vi "FPGA Main v0.2z.vi"() -> ()   [LabVIEW 2021]
uses:
  <vilib>/rvi/Emulation/niFpgaGetClockAttributes.vi
  <vilib>/rvi/Emulation/niFpgaSctlEmulationGetInTimedLoop.vi
  <vilib>/rvi/Emulation/niFpgaEmulationReportErrorSimple.vi
  <vilib>/rvi/eio/common/nirviEmuTemplateMethod_errors.vi
  <vilib>/rvi/Emulation/niFpgaCriticalErrorInLSC.vi
  <vilib>/eio/EIONode/EIONode.xnode
  <vilib>/rvi/FXPMathLib/FxpSub/XNode/nifxpmath_Sub.xnode
  <vilib>/rvi/FXPMathLib/sim/FxpSim.dll
panel:
  in  "DO 1":T1
  out "DI 2":T2
  out "DI 1":T3
  in  "Loop Time (ms)":u32=1 caption="Count(mSec)"
  in  "Stop Button":bool
  out "AI3":fxp<+/-,27,6> format="%.23g"
  out "AI2":fxp<+/-,27,6> format="%.23g"
  out "AI1":fxp<+/-,27,6> format="%.23g"
  out "AI0":fxp<+/-,27,6> format="%.23g"
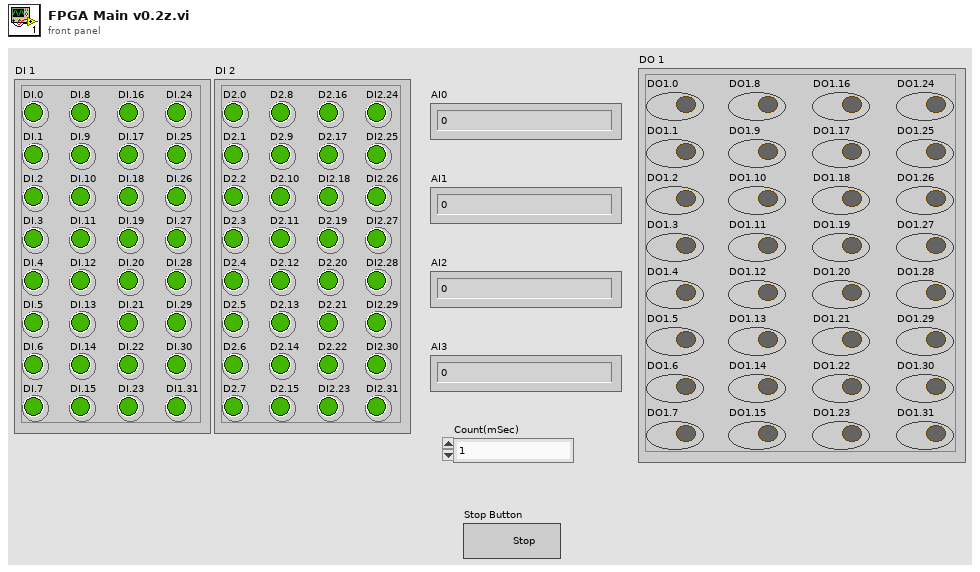
[diagram p1: front panel]
types:
  T1 = cluster{"DO1.0":bool, "DO1.1":bool, "DO1.2":bool, "DO1.3":bool, "DO1.4":bool, "DO1.5":bool, "DO1.6":bool, "DO1.7":bool, "DO1.8":bool, "DO1.9":bool, "DO1.10":bool, "DO1.11":bool, "DO1.12":bool, "DO1.13":bool, "DO1.14":bool, "DO1.15":bool, "DO1.16":bool, "DO1.17":bool, "DO1.18":bool, "DO1.19":bool, "DO1.20":bool, "DO1.21":bool, "DO1.22":bool, "DO1.23":bool, "DO1.24":bool, "DO1.25":bool, "DO1.26":bool, "DO1.27":bool, "DO1.28":bool, "DO1.29":bool, "DO1.30":bool, "DO1.31":bool}
  T2 = cluster{"D2.0 ":bool, "D2.1 ":bool, "D2.2":bool, "D2.3":bool, "D2.4":bool, "D2.5":bool, "D2.6":bool, "D2.7":bool, "D2.8":bool, "D2.9":bool, "D2.10":bool, "D2.11":bool, "D2.12":bool, "D2.13":bool, "D2.14":bool, "D2.15":bool, "D2.16":bool, "D2.17":bool, "DI2.18":bool, "D2.19":bool, "D2.20":bool, "D2.21":bool, "D2.22":bool, "DI2.23":bool, "DI2.24":bool, "DI2.25":bool, "DI2.26":bool, "DI2.27":bool, "DI2.28":bool, "DI2.29":bool, "DI2.30":bool, "DI2.31":bool}
  T3 = cluster{"DI.0":bool, "DI.1 ":bool, "DI.2":bool, "DI.3 ":bool, "DI.4":bool, "DI.5":bool, "DI.6":bool, "DI.7":bool, "DI.8":bool, "DI.9":bool, "DI.10":bool, "DI.11":bool, "DI.12":bool, "DI.13":bool, "DI.14":bool, "DI.15":bool, "DI.16":bool, "DI.17":bool, "DI.18":bool, "DI.19":bool, "DI.20":bool, "DI.21":bool, "DI.22":bool, "DI.23":bool, "DI.24":bool, "DI.25":bool, "DI.26":bool, "DI.27":bool, "DI.28":bool, "DI.29":bool, "DI.30":bool, "DI1.31":bool}
  T4 = cluster{"Boolean array[0]":bool, "Boolean array[1]":bool, "Boolean array[2]":bool, "Boolean array[3]":bool, "Boolean array[4]":bool, "Boolean array[5]":bool, "Boolean array[6]":bool, "Boolean array[7]":bool, "Boolean array[8]":bool, "Boolean array[9]":bool, "Boolean array[10]":bool, "Boolean array[11]":bool, "Boolean array[12]":bool, "Boolean array[13]":bool, "Boolean array[14]":bool, "Boolean array[15]":bool, "Boolean array[16]":bool, "Boolean array[17]":bool, "Boolean array[18]":bool, "Boolean array[19]":bool, "Boolean array[20]":bool, "Boolean array[21]":bool, "Boolean array[22]":bool, "Boolean array[23]":bool, "Boolean array[24]":bool, "Boolean array[25]":bool, "Boolean array[26]":bool, "Boolean array[27]":bool, "Boolean array[28]":bool, "Boolean array[29]":bool, "Boolean array[30]":bool, "Boolean array[31]":bool}
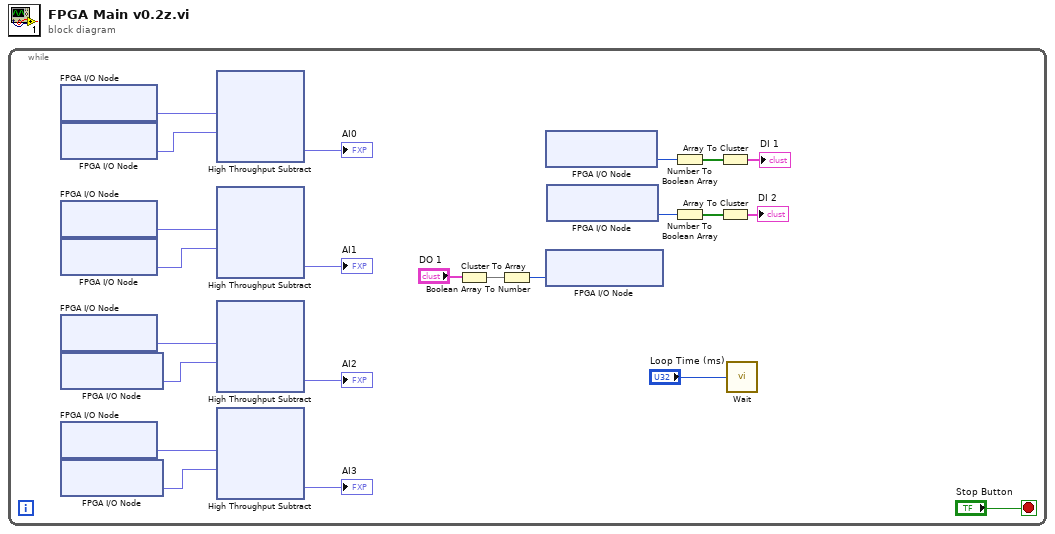
[diagram p0: block diagram]
diagram:
  n1 = while {
    stop <- "Stop Button" stop-if-true
    n2 = xnode "FPGA I/O Node"() -> ("Mod1/AI0"=w23:fxp<+/-,26,5>)  [unwired: 1 in, 1 out]
    n3 = xnode "FPGA I/O Node"() -> ("Mod1/AI8"=w22:fxp<+/-,26,5>)  [unwired: 1 in, 1 out]
    n4 = xnode "FPGA I/O Node"() -> ("Mod1/AI1"=w19:fxp<+/-,26,5>)  [unwired: 1 in, 1 out]
    n5 = xnode "FPGA I/O Node"() -> ("Mod1/AI9"=w18:fxp<+/-,26,5>)  [unwired: 1 in, 1 out]
    n6 = xnode "FPGA I/O Node"() -> ("Mod1/AI2"=w16:fxp<+/-,26,5>)  [unwired: 1 in, 1 out]
    n7 = xnode "FPGA I/O Node"() -> ("Mod1/AI10"=w15:fxp<+/-,26,5>)  [unwired: 1 in, 1 out]
    n8 = xnode "FPGA I/O Node"() -> ("Mod1/AI3"=w13:fxp<+/-,26,5>)  [unwired: 1 in, 1 out]
    n9 = xnode "FPGA I/O Node"() -> ("Mod1/AI11"=w12:fxp<+/-,26,5>)  [unwired: 1 in, 1 out]
    n10 = xnode "High Throughput Subtract"("x"=w23, "y"=w22) -> ("x-y"=→"AI0":fxp<+/-,27,6>)
    n11 = xnode "High Throughput Subtract"("x"=w19, "y"=w18) -> ("x-y"=→"AI1":fxp<+/-,27,6>)
    n12 = xnode "High Throughput Subtract"("x"=w16, "y"=w15) -> ("x-y"=→"AI2":fxp<+/-,27,6>)
    n13 = xnode "High Throughput Subtract"("x"=w13, "y"=w12) -> ("x-y"=→"AI3":fxp<+/-,27,6>)
    n14 = Cluster To Array(cluster="DO 1") -> (array=w3:bool[])
    n15 = Boolean Array To Number(Boolean array=w3) -> (number=w8:u32)
    n16 = xnode "FPGA I/O Node"() -> ("Mod2/DI31:0"=w10:u32)  [unwired: 1 in, 1 out]
    n17 = xnode "FPGA I/O Node"("Mod4/DO31:0"=w8) -> ()  [unwired: 1 in, 1 out]
    n18 = xnode "FPGA I/O Node"() -> ("Mod3/DI31:0"=w9:u32)  [unwired: 1 in, 1 out]
    n19 = Number To Boolean Array(number=w10) -> (Boolean array=w6:bool[])
    n20 = Number To Boolean Array(number=w9) -> (Boolean array=w2:bool[])
    n21 = Array To Cluster(array=w6) -> (cluster=→"DI 1":T4)
    n22 = Array To Cluster(array=w2) -> (cluster=→"DI 2":T4)
    n23 = call "Wait"("Count(mSec)"="Loop Time (ms)") -> ()  [unwired: 1 out]
  }
